vi "Configure External Trigger Source.vi"(8 "error in (no error)":errorcluster, 10 "Trigger Coupling (4: DC)":u16(ring)=4 items=["AC1M", "DC1M", "DC50", "Ground", "DC", "AC", "LFREJ", "HFREJ", "HF"], 11 "VISA resource name":refnum<visa-resource-name>) -> (0 "error out":errorcluster, 3 "VISA resource name out":refnum<visa-resource-name>)   [LabVIEW 2015, in "LeCroy Wave Series.lvlib"]
doc: "Configures external trigger sources. When is used any configure trigger and there select trigger source external, than here you may configure his coupling."
uses:
  <instrlib>/LeCroy Wave Series/LeCroy Wave Series.lvlib
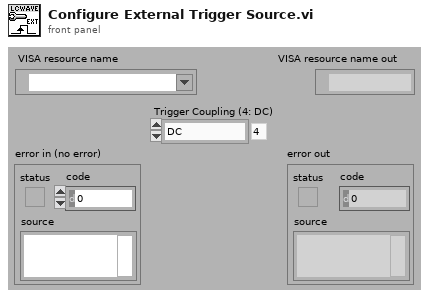
[diagram p1: front panel]
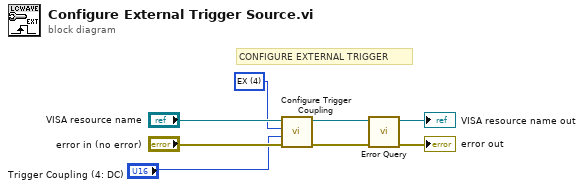
[diagram p0: block diagram]
diagram:
  w2 = u16 4 items=["Channel 1", "Channel 2", "Channel 3", "Channel 4", "EX", "EX10"] ("Channel (0: Channel 1)")
  # "CONFIGURE EXTERNAL TRIGGER"
  n1 = call <instrlib>:"Configure Trigger Coupling.vi"("error in (no error)"="error in (no error)", "Trigger Coupling (4: DC)"="Trigger Coupling (4: DC)", "Trigger Source (0: Channel 1)"=w2, "VISA resource name"="VISA resource name") -> ("error out"=w5:errorcluster, "VISA resource name out"=w6:refnum<visa-resource-name>)  [unwired: 6 in]
  n2 = call <instrlib>:"Error Query.vi"("error in (no error)"=w5, "VISA resource name"=w6) -> ("error out"=→"error out":errorcluster, "VISA resource name out"=→"VISA resource name out":refnum<visa-resource-name>)  [unwired: 6 in, 2 out]
